vi "OP10 Indicators.vi"(8 "error in (no error)":errorcluster, 10 "OUTPUT INDICATOR in":T1, 11 "Boolean in":refnum<vi>) -> (0 "error out":errorcluster, 3 "OUTPUT INDICATOR out":T1)   [LabVIEW 2017]
uses:
  91ced104-a368-4877-bab0-196bafd4c582.vi
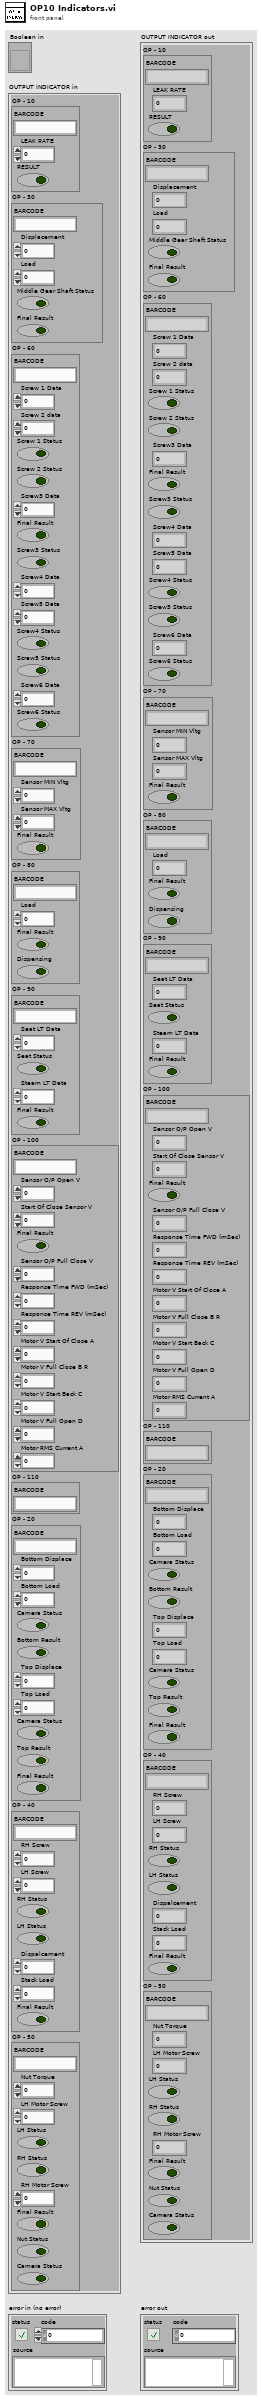
[diagram p1: front panel]
types:
  T1 = cluster{"OP - 10":cluster{"BARCODE":string, "LEAK RATE":dbl, "RESULT":bool}, "OP - 30":cluster{"BARCODE":string, "Displacement":dbl, "Load":dbl, "Middle Gear Shaft Status":bool, "Final Result":bool}, "OP - 60":cluster{"BARCODE":string, "Screw 1 Data":dbl, "Screw 2 data":dbl, "Screw 1 Status":bool, "Screw 2 Status":bool, "Screw3 Data":dbl, "Final Result":bool, "Screw3 Status":bool, "Screw4 Data":dbl, "Screw5 Data":dbl, "Screw4 Status":bool, "Screw5 Status":bool, "Screw6 Data":dbl, "Screw6 Status":bool}, "OP - 70":cluster{"BARCODE":string, "Sensor MIN Vltg":dbl, "Sensor MAX Vltg":dbl, "Final Result":bool}, "OP - 80":cluster{"BARCODE":string, "Load":dbl, "Final Result":bool, "Dispensing":bool}, "OP - 90":cluster{"BARCODE":string, "Seat LT Data":dbl, "Seat Status":bool, "Steam LT Data":dbl, "Final Result":bool}, "OP - 100":cluster{"BARCODE":string, "Sensor O/P Open V":dbl, "Start Of Close Sensor V":dbl, "Final Result":bool, "Sensor O/P Full Close V":dbl, "Response Time FWD (mSec)":dbl, "Response Time REV (mSec)":dbl, "Motor V Start Of Close A":dbl, "Motor V Full Close B R":dbl, "Motor V Start Back C":dbl, "Motor V Full Open D":dbl, "Motor RMS Current A":dbl}, "OP - 110":cluster{"BARCODE":string}, "OP - 20":cluster{"BARCODE":string, "Bottom Displace":dbl, "Bottom Load":dbl, "Camera Status":bool, "Bottom Result":bool, "Top Displace":dbl, "Top Load ":dbl, "Camera Status":bool, "Top Result":bool, "Final Result":bool}, "OP - 40":cluster{"BARCODE":string, "RH Screw":dbl, "LH Screw ":dbl, "RH Status":bool, "LH Status":bool, "Dispalcement ":dbl, "Stack Load ":dbl, "Final Result":bool}, "OP - 50":cluster{"BARCODE":string, "Nut Torque":dbl, "LH Motor Screw":dbl, "LH Status":bool, "RH Status":bool, "RH Motor Screw":dbl, "Final Result":bool, "Nut Status":bool, "Camera Status":bool}}
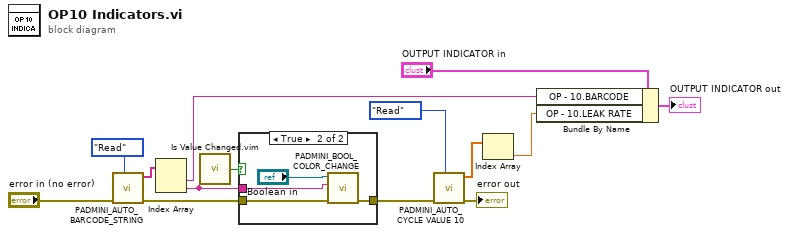
[diagram p0: block diagram]
diagram:
  n1 = call "PADMINI_AUTO_BARCODE_STRING.vi"("Enum"=enum16{"Read", "Write"}."Read", "error in (no error)"="error in (no error)") -> ("error out"=w9:errorcluster, "Input 2"=w2:string[])  [unwired: 8 in]
  n2 = Index Array(array=w2) -> (element #1=w4:string, element #2=w10:string)  [unwired: 2 in]
  n3 = call "Is Value Changed.vim"("value"=w10) -> ("changed or first call?"=w12:bool)
  n4 = case shown="True" w12 {
    tunnel: [w15 w19] -> w7
    tunnel: w10 -> [_ w18]
    tunnel: w9 -> [w15 w17]
    frame False {
    }
    frame True {
      n5 = call "PADMINI_BOOL_COLOR_CHANGE.vi"("error in (no error)"=w17, "Input Result"=w18, "Boolean in"="Boolean in") -> ("error out"=w19:errorcluster)  [unwired: 8 in]
    }
  }
  n6 = call "PADMINI_AUTO_CYCLE VALUE 10.vi"("Enum"=enum16{"Read", "Write"}."Read", "error in (no error)"=w7) -> ("error out"=→"error out":errorcluster, "Input 2"=w6:sgl[])  [unwired: 8 in]
  n7 = Index Array(array=w6) -> (element=w8:sgl)  [unwired: 1 in]
  n8 = Bundle By Name(cluster="OUTPUT INDICATOR in", "OP - 10.BARCODE"=w4, "OP - 10.LEAK RATE"=w8) -> (→"OUTPUT INDICATOR out":T1)
